vi "Obtain Session.vi"(0 "SequenceFile":refnum<k7>, 2 "Engine":T1, 11 "error in (no error)":errorcluster) -> (4 "Session Handle":T2, 15 "error out":errorcluster)   [LabVIEW 2019, in "HTS.lvlib" / "SequenceFile.lvclass"]
doc: "This function initializes the measurement\n\nPass the function a name to obtain an active measurement handle"
uses:
  SequenceFile.lvclass
  Program Files (x86)/National Instruments/LabVIEW 2020/user.lib/_Session Fwk/Session - Root.lvclass
  Typedefs/Session Handle.ctl
  Engine/Engine.lvclass
  Engine/Typedefs/Session Handle.ctl
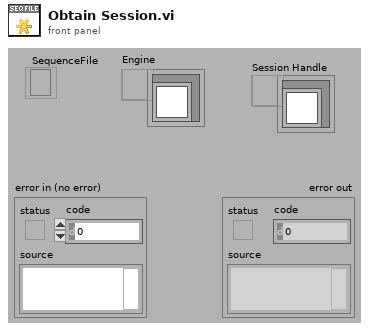
[diagram p1: front panel]
types:
  T1 = typedef "HTS.lvlib/Engine.lvclass/Session Handle.ctl" = refnum<data-value>
  T2 = typedef "HTS.lvlib/SequenceFile.lvclass/Session Handle.ctl" = refnum<data-value>
  T3 = typedef "Session - Root.lvclass/Session Handle.ctl" = refnum<data-value>
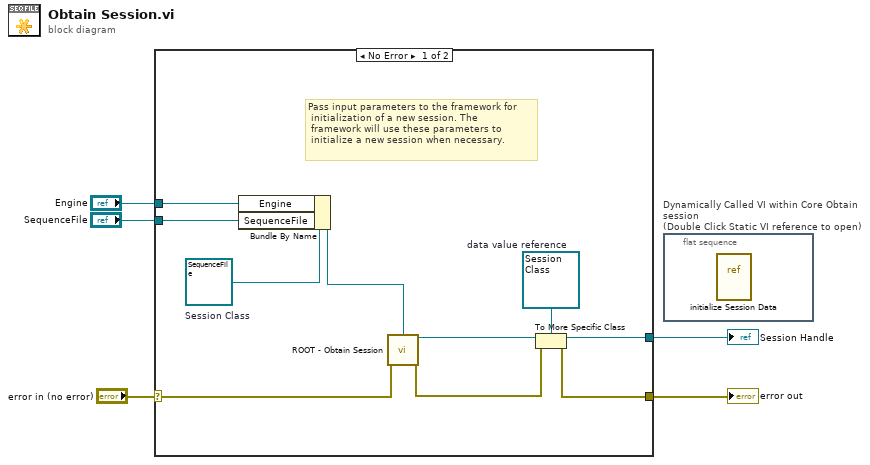
[diagram p0: block diagram]
diagram:
  n1 = case shown="No Error" "error in (no error)" {
    selector: "error in (no error)" -> [w15 w16]
    tunnel: [w12 w16] -> w4
    tunnel: [w14 _] -> w3
    tunnel: "SequenceFile" -> [w7 _]
    tunnel: "Engine" -> [w6 _]
    frame No Error {
      w8 = refnum<data-value> refnum  # data value reference
      w9 = refnum<class "SequenceFile.lvclass"> refnum  # Session Class
      # "Pass input parameters to the framework for\n initialization of a new session. The\n framework will use these parameters to\n initialize a new session when necessary."
      n2 = Bundle By Name(cluster=w9, "Engine"=w6, "SequenceFile"=w7) -> (w10:refnum<class "SequenceFile.lvclass">)
      n3 = call "ROOT - Obtain Session.vi"("OBJ - Session"=w10, "error in (no error)"=w15) -> ("Session Handle"=w11:T3, "error out"=w13:errorcluster)  [unwired: 11 in, 1 out]
      n4 = To More Specific Class(target class=w8, reference=w11, error in=w13) -> (specific class reference=w14:refnum<data-value>, error out=w12:errorcluster)
    }
    frame Error {
    }
  }
  "error out" <- w4
  "Session Handle" <- w3
  n5 = flat-sequence "Dynamically Called VI within Core Obtain session\n(Double Click Static VI reference to open)" {
    frame #0 {
      n6 = vi-ref "initialize Session Data.vi"() -> ()  [unwired: 1 out]
    }
  }
